vi "校准信息改变发送 (子VI).vi"(8 "错误输入":errorcluster caption="错误输出") -> (0 "错误输出":errorcluster)   [LabVIEW 2016, in "数据传输系统-06.lvlib"]
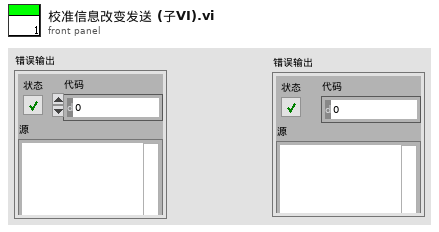
[diagram p1: front panel]
types:
  T1 = cluster{"低标液1浓度":dbl, "低标液1信号值":dbl, "低标液1启用":u16, "低标液2浓度":dbl, "低标液2信号值":dbl, "低标液2启用":u16, "低标液3浓度":dbl, "低标液3信号值":dbl, "低标液3启用":u16, "低标液4浓度":dbl, "低标液4信号值":dbl, "低标液4启用":u16, "低标液5浓度":dbl, "低标液5信号值":dbl, "低标液5启用":u16, "高标液1浓度":dbl, "高标液1信号值":dbl, "高标液1启用":u16, "高标液2浓度":dbl, "高标液2信号值":dbl, "高标液2启用":u16, "高标液3浓度":dbl, "高标液3信号值":dbl, "高标液3启用":u16, "高标液4浓度":dbl, "高标液4信号值":dbl, "高标液4启用":u16, "高标液5浓度":dbl, "高标液5信号值":dbl, "高标液5启用":u16, "低斜率":dbl, "低截距":dbl, "低二次多项式系数":dbl, "低线性相关系数":dbl, "高斜率":dbl, "高截距":dbl, "高二次多项式系数":dbl, "高线性相关系数":dbl}
  T2 = cluster{"CODMn校准信息":bool, "氨氮校准信息":bool, "总磷校准信息":bool, "总氮校准信息":bool, "CODCr校准信息":bool}
  T3 = cluster{"低标液1浓度":dbl, "低标液1信号值":dbl, "低标液1启用":u16, "低标液2浓度":dbl, "低标液2信号值":dbl, "低标液2启用":u16, "低标液3浓度":dbl, "低标液3信号值":dbl, "低标液3启用":u16, "低标液4浓度":dbl, "低标液4信号值":dbl, "低标液4启用":u16, "低标液5浓度":dbl, "低标液5信号值":dbl, "低标液5启用":u16, "高标液1浓度":dbl, "高标液1信号值":dbl, "高标液1启用":u16, "高标液2浓度":dbl, "高标液2信号值":dbl, "高标液2启用":u16, "高标液3浓度":dbl, "高标液3信号值":dbl, "高标液3启用":u16, "高标液4浓度":dbl, "高标液4信号值":dbl, "高标液4启用":u16, "高标液5浓度":dbl, "高标液5信号值":dbl, "高标液5启用":u16, "低斜率":dbl, "低截距":dbl, "低二次多项式系数":dbl, "低线性相关系数":dbl, "高斜率":dbl, "高截距":dbl, "高二次多项式系数":dbl, "高线性相关系数":dbl}[]
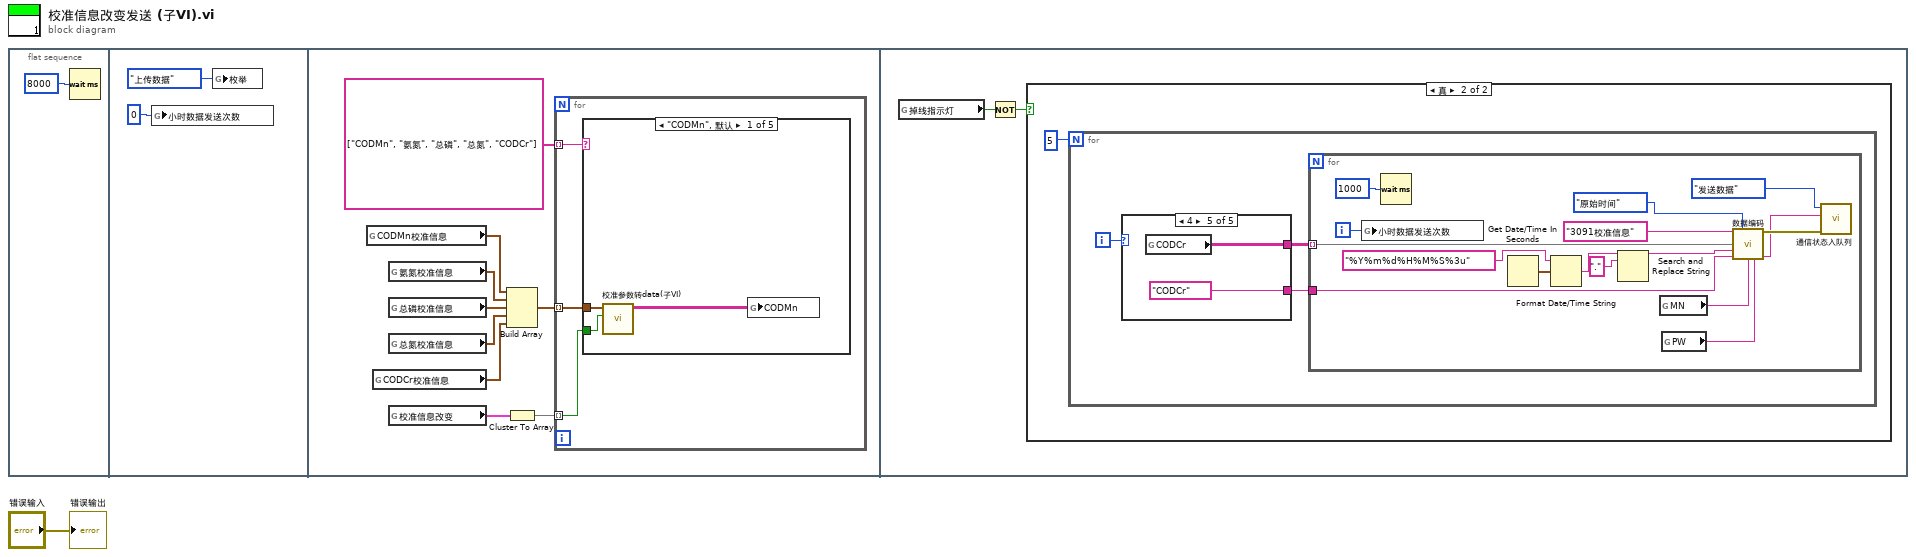
[diagram p0: block diagram]
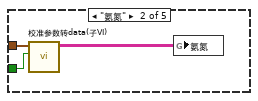
[diagram p2: hidden frame]
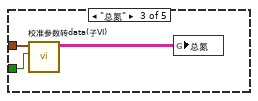
[diagram p3: hidden frame]
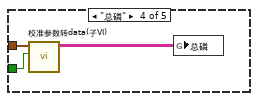
[diagram p4: hidden frame]
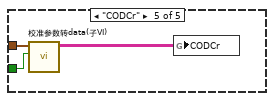
[diagram p5: hidden frame]
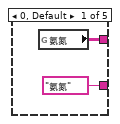
[diagram p7: hidden frame]
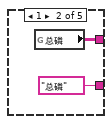
[diagram p8: hidden frame]
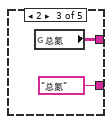
[diagram p9: hidden frame]
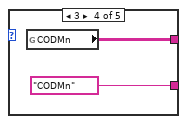
[diagram p10: hidden frame]
diagram:
  n1 = flat-sequence {
    frame #0 {
      n2 = Wait (ms)(milliseconds to wait=u32 8000 ("等待时间（毫秒）")) -> ()  [unwired: 1 out]
    }
    frame #1 {
      n3 = global write "全局 小时数据发送次数.vi" "小时数据发送次数"(0 ("小时数据发送次数")) -> ()
      n4 = global write "全局1.vi" "枚举"(enum16{"返回请求应答", "上传数据", "返回执行结果"}."上传数据" ("枚举")) -> ()
    }
    frame #2 {
      n5 = global read "全局1.vi" "CODMn校准信息"() -> (w10:T1)
      n6 = global read "全局1.vi" "CODCr校准信息"() -> (w13:T1)
      n7 = global read "全局1.vi" "氨氮校准信息"() -> (w12:T1)
      n8 = global read "全局1.vi" "总磷校准信息"() -> (w8:T1)
      n9 = global read "全局1.vi" "总氮校准信息"() -> (w7:T1)
      n10 = global read "全局1.vi" "校准信息改变"() -> (w6:T2)
      n11 = Build Array(w10, w12, w8, w7, w13) -> (w11:T3)
      n12 = Cluster To Array(cluster=w6) -> (array=w5:bool[])
      n13 = for {
        tunnel: string[] ["CODMn", "氨氮", "总磷", "总氮", "CODCr"] -> [w16] mode=indexing
        tunnel: w11 -> [w15] mode=indexing
        tunnel: w5 -> [w14] mode=indexing
        n14 = case shown="\"CODMn\", 默认" w16 {
          tunnel: w15 -> [w19 w22 w25 w28 w31]
          tunnel: w14 -> [w18 w21 w24 w27 w30]
          frame "CODMn", Default {
            n15 = call "校准参数转data(子VI).vi"("改变?"=w18, "校准信息"=w19) -> ("数组"=w17:string[][])  [unwired: 9 in]
            n16 = global write "全局 所有参数.vi" "CODMn"(w17) -> ()
          }
          frame "氨氮" {
            n17 = call "校准参数转data(子VI).vi"("改变?"=w21, "校准信息"=w22) -> ("数组"=w20:string[][])  [unwired: 9 in]
            n18 = global write "全局 所有参数.vi" "氨氮"(w20) -> ()
          }
          frame "总氮" {
            n19 = call "校准参数转data(子VI).vi"("改变?"=w24, "校准信息"=w25) -> ("数组"=w23:string[][])  [unwired: 9 in]
            n20 = global write "全局 所有参数.vi" "总氮"(w23) -> ()
          }
          frame "总磷" {
            n21 = call "校准参数转data(子VI).vi"("改变?"=w27, "校准信息"=w28) -> ("数组"=w26:string[][])  [unwired: 9 in]
            n22 = global write "全局 所有参数.vi" "总磷"(w26) -> ()
          }
          frame "CODCr" {
            n23 = call "校准参数转data(子VI).vi"("改变?"=w30, "校准信息"=w31) -> ("数组"=w29:string[][])  [unwired: 9 in]
            n24 = global write "全局 所有参数.vi" "CODCr"(w29) -> ()
          }
        }
      }
    }
    frame #3 {
      n25 = global read "全局 数据发送重叠.vi" "掉线指示灯"() -> (w33:bool)
      n26 = Not(x=w33) -> (.not. x?=w32:bool)
      n27 = case shown="真" w32 {
        frame False {
        }
        frame True {
          n28 = for {
            N: 5 -> [_]
            i -> [w37]
            n29 = case shown="4" w37 {
              tunnel: [w39 w41 w43 w45 w47] -> w36
              tunnel: ["氨氮" ("污染物编码") "总磷" ("污染物编码") "总氮" ("污染物编码") "CODMn" ("污染物编码") "CODCr" ("污染物编码")] -> w35
              frame 0, Default {
                n30 = global read "全局 所有参数.vi" "氨氮"() -> (w39:string[][])
              }
              frame 1 {
                n31 = global read "全局 所有参数.vi" "总磷"() -> (w41:string[][])
              }
              frame 2 {
                n32 = global read "全局 所有参数.vi" "总氮"() -> (w43:string[][])
              }
              frame 3 {
                n33 = global read "全局 所有参数.vi" "CODMn"() -> (w45:string[][])
              }
              frame 4 {
                n34 = global read "全局 所有参数.vi" "CODCr"() -> (w47:string[][])
              }
            }
            n35 = for {
              tunnel: w35 -> [w63]
              tunnel: w36 -> [w62] mode=indexing
              i -> [w61]
              n36 = global write "全局 小时数据发送次数.vi" "小时数据发送次数"(w61) -> ()
              n37 = Wait (ms)(milliseconds to wait=u32 1000 ("等待时间（毫秒）")) -> ()  [unwired: 1 out]
              n38 = Get Date/Time In Seconds() -> (seconds since 1Jan1904=w58:timestamp)
              n39 = Format Date/Time String(time format string (%c)="%Y%m%d%H%M%S%3u" ("时间格式字符串(%c)"), seconds (now)=w58) -> (date/time string=w57:string)  [unwired: 1 in]
              n40 = Search and Replace String(input string=w57, search string="." ("搜索字符串")) -> (result string=w55:string)  [unwired: 6 in, 3 out]
              n41 = global read "断电保存全局.vi" "MN"() -> (w54:string)
              n42 = global read "断电保存全局.vi" "PW"() -> (w53:string)
              n43 = call "数据编码.vi"("table输入"="3091校准信息" ("新元素/子数组"), "仪器参数上传时间"=enum16{"精确到小时", "原始时间"}."原始时间", "仪器参数"=w62, "QN"=w55, "参数"=w63, "MN"=w54, "PW"=w53) -> ("错误常量"=w52:errorcluster, "通讯包字符串"=w48:string)  [unwired: 7 in]
              n44 = call "通信状态入队列.vi"("错误输入（无错误）"=w52, "发送报文"=w48, "枚举"=enum16{"打开连接", "发送数据", "读取数据", "数据处理", "关闭连接"}."发送数据") -> ()  [unwired: 8 in, 1 out]
            }
          }
        }
      }
    }
  }
  "错误输出" <- "错误输入"
